vi "System Status Management Core.vi"(11 "CIFPluginManager in":refnum<class "CIFPluginManager.lvclass">) -> (0 "error out":errorcluster)   [LabVIEW 2021, in "CIFPluginManager.lvclass"]
uses:
  CIFPluginManager.lvclass
  CIFPluginManager.lvclass/CIFPluginManager.ctl
  gRPC/CIF_Manager_server/RPC Service/Manager/Manager.lvclass
  C:/Program Files/National Instruments/LabVIEW 2021/vi.lib/gRPC/LabVIEW gRPC Servicer/ServiceBase/ServiceBase.lvclass
  gRPC/CIF_Manager_server/RPC Service/Manager/Manager.lvclass/Manager.ctl
  gRPC/CIF_Manager_server/RPC Messages/cif_manager_QuerySystemStatusResponse.ctl
  gRPC/CIF_Manager_server/RPC Messages/cif_manager_SystemStatus.ctl
  gRPC/CIF_Manager_server/RPC Messages/cif_manager_ClockConversionArray.ctl
  gRPC/CIF_Manager_server/RPC Messages/cif_manager_ClockConversion.ctl
  gRPC/CIF_Manager_server/RPC Messages/cif_manager_TimePair.ctl
  gRPC/CIF_Manager_server/RPC Messages/Get cif_manager_QuerySystemStatusRequest.vi
  gRPC/CIF_Manager_server/RPC Messages/Set cif_manager_QuerySystemStatusResponse.vi
  gRPC/CIF_Manager_server/RPC Messages/Get cif_manager_QuerySystemStatusRequest.vi/2ed25e12-861d-4677-8ead-ace2906b2041.vi
  gRPC/CIF_Manager_server/RPC Messages/FlatToRichcif_manager_QuerySystemStatusRequest.vi
  gRPC/CIF_Manager_server/RPC Messages/Set cif_manager_QuerySystemStatusResponse.vi/dcc74a39-081a-4bdd-860b-8ed792803c96.vi
  gRPC/CIF_Manager_server/RPC Messages/RichToFlatcif_manager_QuerySystemStatusResponse.vi
  <vilib>/gRPC/LabVIEW gRPC Library/Shared/TranslateGrpcError.vi
  gRPC/CIF_Manager_server/RPC Messages/FlatToRichcif_manager_PluginStatus.vi
  gRPC/CIF_Manager_server/RPC Messages/RichToFlatcif_manager_SystemStatus.vi
  gRPC/CIF_Manager_server/RPC Messages/FlatToRichcif_management_common_PluginStatusData.vi
  gRPC/CIF_Manager_server/RPC Messages/FlatToRichcif_management_common_Channels.vi
  gRPC/CIF_Manager_server/RPC Messages/RichToFlatcif_manager_ClockConversionArray.vi
  gRPC/CIF_Manager_server/RPC Messages/FlatToRichcif_management_common_TimingStatistics.vi
  gRPC/CIF_Manager_server/RPC Messages/FlatToRichcif_management_common_FifoStatistics.vi
  gRPC/CIF_Manager_server/RPC Messages/FlatToRichcif_management_common_Error.vi
  gRPC/CIF_Manager_server/RPC Messages/FlatToRichcif_management_common_MonitorDoubles.vi
  gRPC/CIF_Manager_server/RPC Messages/FlatToRichcif_management_common_MonitorU64.vi
  gRPC/CIF_Manager_server/RPC Messages/FlatToRichcif_management_common_MonitorI64.vi
  gRPC/CIF_Manager_server/RPC Messages/FlatToRichcif_management_common_Channel.vi
  gRPC/CIF_Manager_server/RPC Messages/RichToFlatcif_manager_ClockConversion.vi
  gRPC/CIF_Manager_server/RPC Messages/FlatToRichcif_common_TimingStats.vi
  gRPC/CIF_Manager_server/RPC Messages/RichToFlatcif_manager_TimePair.vi
  <vilib>/gRPC/LabVIEW gRPC Library/Server API/Server/Get Server DLL Path.vi
  <vilib>/Utility/error.llb/Error Cluster From Error Code.vi
  <vilib>/gRPC/LabVIEW gRPC Library/Server API/Message Requests/Complete Call.vi
  <vilib>/CIF Foundation/CIF Core/CIFUtilities/CIFLogs/CIFLogs.lvlib
  gRPC/CIF_Manager_server/CIF_Manager_server.lvlib
  <vilib>/CIF Foundation/CIF Utilities/Time/Time_CIF_U.lvlib
  <vilib>/CIF Foundation/CIF Core/CIFPluginManager/gRPC/CIF_Manager_Client_Wrapper/CIFManagerClientWrapper.lvlib
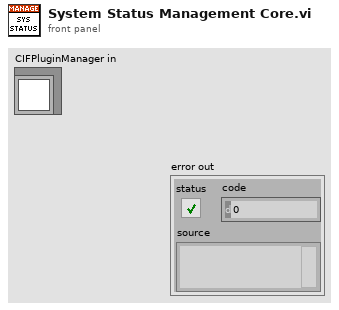
[diagram p1: front panel]
types:
  T1 = typedef "CIF_Manager_server.lvlib/Manager.lvclass/Server gRPC UEs.ctl" = cluster{"Manager LoadPlugin gRPC UE":refnum<user-event>, "Manager RegisterPlugin gRPC UE":refnum<user-event>, "Manager UnregisterPlugin gRPC UE":refnum<user-event>, "Manager QueryPluginTypes gRPC UE":refnum<user-event>, "Manager AbortPlugin gRPC UE":refnum<user-event>, "Manager UnloadAllPlugins gRPC UE":refnum<user-event>, "Manager Destroy gRPC UE":refnum<user-event>, "Manager Ping gRPC UE":refnum<user-event>, "Manager QueryErrors gRPC UE":refnum<user-event>, "Manager QueryConfig gRPC UE":refnum<user-event>, "Manager QueryInfo gRPC UE":refnum<user-event>, "Manager ResetErrorIndex gRPC UE":refnum<user-event>, "Manager ResetConfigIndex gRPC UE":refnum<user-event>, "Manager ResetInfoIndex gRPC UE":refnum<user-event>, "Manager QueryPluginInfo gRPC UE":refnum<user-event>, "Manager QueryPlugin gRPC UE":refnum<user-event>, "Manager QuerySystemStatus gRPC UE":refnum<user-event>, "Manager UpdateClock gRPC UE":refnum<user-event>, "Manager CreateOrch gRPC UE":refnum<user-event>, "Manager QueryClockStatus gRPC UE":refnum<user-event>, "Manager QueryAllChannels gRPC UE":refnum<user-event>, "Manager RegisterPluginLoader gRPC UE":refnum<user-event>, "Manager UnregisterPluginLoader gRPC UE":refnum<user-event>, "Manager CreatePluginLoader gRPC UE":refnum<user-event>, "Manager DestroyPluginLoader gRPC UE":refnum<user-event>, "Manager QueryPluginLoaders gRPC UE":refnum<user-event>}
  T2 = typedef "CIF_Manager_server.lvlib/cif_manager_QuerySystemStatusResponse.ctl" = cluster{"system_status":T3}
  T3 = typedef "CIF_Manager_server.lvlib/cif_manager_SystemStatus.ctl" = cluster{"clock_conversion_array":T4}
  T4 = typedef "CIF_Manager_server.lvlib/cif_manager_ClockConversionArray.ctl" = cluster{"clock_conversions":T5[]}
  T5 = typedef "CIF_Manager_server.lvlib/cif_manager_ClockConversion.ctl" = cluster{"clock_id":u32, "last_reset":i64, "slope":dbl, "offset_pair":T6, "clock_name":string}
  T6 = typedef "CIF_Manager_server.lvlib/cif_manager_TimePair.ctl" = cluster{"system_time":i64, "external_time":i64}
  T7 = typedef "grpc-lvsupport-release.lvlib/grpcId.ctl" = u64
  T8 = typedef "CIF_Manager_server.lvlib/cif_manager_QuerySystemStatusRequest.ctl" = cluster{"plugin_status":T9}
  T9 = typedef "CIF_Manager_server.lvlib/cif_manager_PluginStatus.ctl" = cluster{"pluginname":string, "status":T10, "channels":T19}
  T10 = typedef "CIF_Manager_server.lvlib/cif_management_common_PluginStatusData.ctl" = cluster{"state":T11, "timing_statistics":T12, "fifo_statistics":T14, "error":T15, "monitor_doubles":T16, "monitor_u64s":T17, "monitor_i64s":T18}
  T11 = typedef "CIF_Manager_server.lvlib/cif_management_common_PluginStatusData_PluginState.ctl" = enum32{"PLUGINSTATE_UNKNOWN", "PLUGINSTATE_CREATING", "PLUGINSTATE_LISTENING", "PLUGINSTATE_RUNNING", "PLUGINSTATE_CLEANINGUP", "PLUGINSTATE_DESTROYING"}
  T12 = typedef "CIF_Manager_server.lvlib/cif_management_common_TimingStatistics.ctl" = cluster{"period":T13, "wake_error":T13, "execute":T13, "housekeep":T13, "idle":T13, "cleanup":T13, "custom_1":T13, "custom_2":T13}
  T13 = typedef "CIF_Manager_server.lvlib/cif_common_TimingStats.ctl" = cluster{"max":i64, "min":i64, "avg":dbl}
  T14 = typedef "CIF_Manager_server.lvlib/cif_management_common_FifoStatistics.ctl" = cluster{"from_t0":T13, "from_previous_plugin":T13, "output_error":T13}
  T15 = typedef "CIF_Manager_server.lvlib/cif_management_common_Error.ctl" = cluster{"status":bool, "code":i32}
  T16 = typedef "CIF_Manager_server.lvlib/cif_management_common_MonitorDoubles.ctl" = cluster{"double_1":dbl, "double_2":dbl, "double_3":dbl, "double_4":dbl}
  T17 = typedef "CIF_Manager_server.lvlib/cif_management_common_MonitorU64.ctl" = cluster{"u64_1":u64, "u64_2":u64, "u64_3":u64, "u64_4":u64}
  T18 = typedef "CIF_Manager_server.lvlib/cif_management_common_MonitorI64.ctl" = cluster{"i64_1":i64, "i64_2":i64, "i64_3":i64, "i64_4":i64}
  T19 = typedef "CIF_Manager_server.lvlib/cif_management_common_Channels.ctl" = cluster{"channels":T20[]}
  T20 = typedef "CIF_Manager_server.lvlib/cif_management_common_Channel.ctl" = cluster{"name":string, "direction":T21, "type":string, "custom_config":u8[], "connected":bool, "connected_name":string, "forced":bool, "channel_pattern":T22}
  T21 = typedef "CIF_Manager_server.lvlib/cif_management_common_ChannelDirection.ctl" = enum32{"CHANNELDIRECTION_UNKNOWN", "CHANNELDIRECTION_PUBLISHER", "CHANNELDIRECTION_SUBSCRIBER"}
  T22 = typedef "CIF_Manager_server.lvlib/cif_management_common_ChannelPattern.ctl" = enum32{"CHANNELPATTERN_UNKNOWN", "CHANNELPATTERN_TAG", "CHANNELPATTERN_FIFO", "CHANNELPATTERN_MULTIFIFO", "CHANNELPATTERN_BACKPRESSUREFIFO"}
  T23 = typedef "Time_CIF_U.lvlib/Clock History Map.ctl" = map{u8, T24}
  T24 = typedef "Time_CIF_U.lvlib/Clock History.ctl" = cluster{"System Clock":i64[], "External Clock":i64[], "Last Reset Time":i64, "slope":dbl, "1/slope":dbl, "Offset Pair":T25, "Name":string}
  T25 = typedef "Time_CIF_U.lvlib/Timestamp Pair.ctl" = cluster{"System Time":i64, "External Time":i64}
  T26 = typedef "Time_CIF_U.lvlib/Clock Conversion.ctl" = cluster{"ClockID":u8, "Last Reset":i64, "Offset Pair":T25, "Slope":dbl, "1/Slope":dbl, "Name":string}
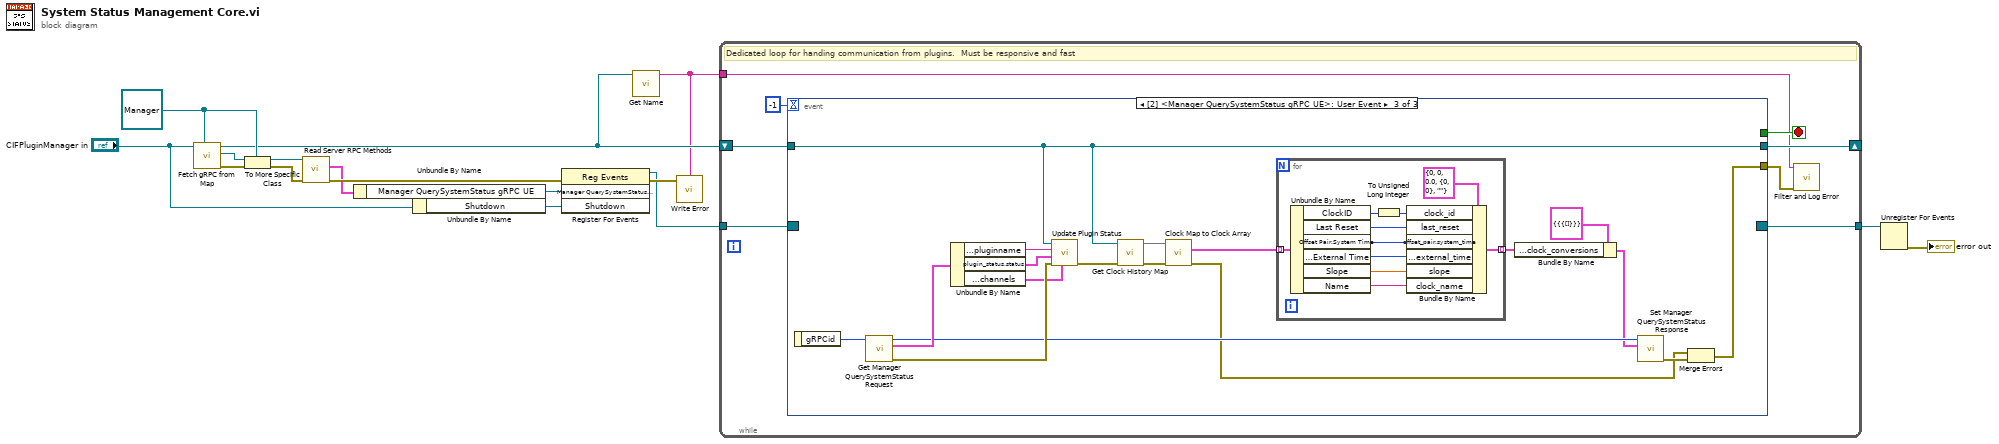
[diagram p0: block diagram]
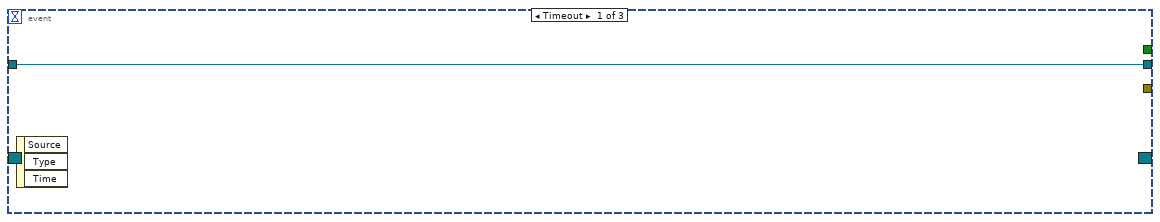
[diagram p2: hidden frame]
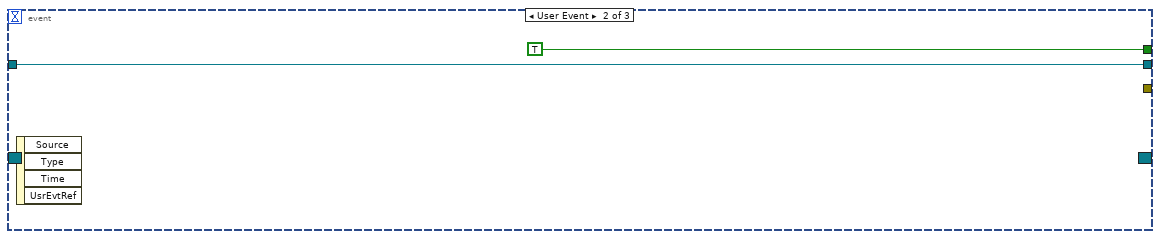
[diagram p3: hidden frame]
diagram:
  w13 = refnum<class "Manager.lvclass"> refnum ("CIF_Manager_server.lvlib:Manager.lvclass")
  n1 = call "Fetch gRPC from Map.vi"("gRPC Server Class type"=w13, "Plugin Manager in"="CIFPluginManager in") -> ("error out"=w12:errorcluster, "gRPC Server Class out"=w14:refnum<class "ServiceBase.lvclass">, "Plugin Manager out"=w2:refnum<class "CIFPluginManager.lvclass">)  [unwired: 7 in]
  n2 = To More Specific Class(target class=w13, reference=w14, error in=w12) -> (specific class reference=w10:refnum<class "Manager.lvclass">, error out=w11:errorcluster)
  n3 = call "Read Server RPC Methods.vi"("error in (no error)"=w11, "gRPC service in"=w10) -> ("error out"=w5:errorcluster, "Server RPC Methods"=w4:T1)  [unwired: 7 in, 1 out]
  n4 = Unbundle By Name(w4) -> ("Manager QuerySystemStatus gRPC UE"=w3:refnum<user-event>)
  n5 = Unbundle By Name("CIFPluginManager in") -> ("Shutdown"=w9:refnum<user-event>)
  n6 = register-events(error in=w5, w3, w9) -> (reference out=w6:refnum<event-registration>, error out=w7:errorcluster)  [unwired: 1 in]
  n7 = call "Get Name.vi"("CIFPluginManager in"=w2) -> ("Name"=w1:string)  [unwired: 10 in]
  n8 = call <vilib>:"Write Error.vi"("error in (no error)"=w7, "Plugin Name"=w1) -> ()  [unwired: 2 in, 1 out]
  n9 = while {
    tunnel: w6 -> [w24]
    shift-right: [w19] -> _
    shift-left: w2 -> [w23]
    tunnel: [w20] -> w15
    tunnel: w1 -> [w17]
    stop <- w21 stop-if-true
    # "Dedicated loop for handing communication from plugins.  Must be responsive and fast"
    n10 = event shown="[2] <Manager QuerySystemStatus gRPC UE>: User Event" {
      selector: w24 -> [_ _ _]
      dyn-events: [_ _ _] -> w20
      timeout: -1 -> [_ _ _]
      tunnel: w23 -> [w25 w26 w31]
      tunnel: [_ TRUE _] -> w21
      tunnel: [_ _ w36] -> w18
      tunnel: [w25 w26 w31] -> w19
      event Timeout {
        n11 = event-data() -> ()  [unwired: 1 in, 3 out]
      }
      event User Event {
        n12 = event-data() -> ()  [unwired: 1 in, 4 out]
      }
      event User Event {
        n13 = event-data() -> ("gRPCid"=w37:T7)  [unwired: 1 in]
        n14 = call "Get Manager QuerySystemStatus Request.vi"("gRPCid"=w37) -> ("error out"=w44:errorcluster, "Message Data"=w41:T8, "gRPCid out"=w38:T7)  [unwired: 8 in]
        n15 = Unbundle By Name(w41) -> ("plugin_status.pluginname"=w42:string, "plugin_status.status"=w43:T10, "plugin_status.channels"=w30:T19)
        n16 = call "Update Plugin Status.vi"("channels"=w30, "error in (no error)"=w44, "Status"=w43, "Plugin Name"=w42, "Launcher in"=w31) -> ("error out"=w34:errorcluster)  [unwired: 6 in]
        n17 = call "Get Clock History Map.vi"("error in (no error)"=w34, "CIFPluginManager in"=w31) -> ("error out"=w33:errorcluster, "Clock History Map"=w35:T23)  [unwired: 8 in]
        n18 = call <vilib>:"Clock Map to Clock Array.vi"("error in (no error)"=w33, "Clock History Map in"=w35) -> ("error out"=w32:errorcluster, "Clock Conversion Array"=w45:T26[])  [unwired: 7 in, 1 out]
        n19 = for {
          tunnel: w45 -> [w54] mode=indexing
          tunnel: [w46] -> w40 mode=indexing
          n20 = Unbundle By Name(w54) -> ("ClockID"=w53:u8, "Last Reset"=w47:i64, "Offset Pair.System Time"=w48:i64, "Offset Pair.External Time"=w49:i64, "Slope"=w50:dbl, "Name"=w51:string)
          n21 = To Unsigned Long Integer(number=w53) -> (unsigned 32bit integer=w52:u32)
          n22 = Bundle By Name(cluster=T5 {"clock_id"=0, "last_reset"=0, "slope"=0.0, "offset_pair"={"system_time"=0, "external_time"=0}, "clock_name"=""} ("cif_manager_ClockConversion"), "clock_id"=w52, "last_reset"=w47, "offset_pair.system_time"=w48, "offset_pair.external_time"=w49, "slope"=w50, "clock_name"=w51) -> (w46:T5)
        }
        n23 = Bundle By Name(cluster=T2 {"system_status"={"clock_conversion_array"={"clock_conversions"=[]}}} ("Message Data"), "system_status.clock_conversion_array.clock_conversions"=w40) -> (w28:T2)
        n24 = call "Set Manager QuerySystemStatus Response.vi"("Message Data"=w28, "gRPCid in"=w38) -> ("error out"=w39:errorcluster)  [unwired: 9 in]
        n25 = Merge Errors(w32, w39) -> (w36:errorcluster)
      }
    }
    n26 = call <vilib>:"Filter and Log Error.vi"("error In"=w18, "Name"=w17) -> ()  [unwired: 10 in]
  }
  n27 = Unregister For Events(event registration refnum=w15) -> (error out=→"error out":errorcluster)  [unwired: 1 in]
